vi "Perform Action.vi"(8 "error in":errorcluster, 10 "Input":variant, 11 "HSU MCU V2 in":refnum<class "HSU MCU V2 CFG.lvclass">) -> (0 "error out":errorcluster, 2 "Output":variant, 3 "HSU MCU V2 out":refnum<class "HSU MCU V2 CFG.lvclass">)   [LabVIEW 2023, in "HSU MCU V2 CFG.lvclass"]
uses:
  HSU MCU V2 CFG.lvclass
  Attribute Selector.ctl
  MCU Selector.ctl
  HSU MCU V2 CFG.lvclass/HSU MCU V2 CFG.ctl
  Protocols/ICAN/ICAN.lvclass
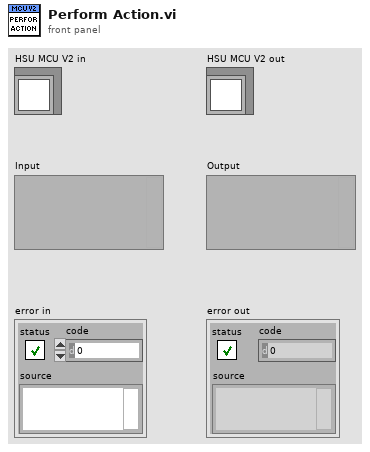
[diagram p1: front panel]
types:
  T1 = typedef "MCU Selector.ctl" = enum16{"Default", "MCU1", "MCU2", "MCU3", "MCU4", "MCU5", "MCU6", "MCU7", "MCU8", "ALL"}
  T2 = typedef "Attribute Selector.ctl" = enum16{"MCU_FAULT", "ALL", "MCU_STATE", "MCU_Temp_Winding", "MCU_Temp_PowerStage", "MCU_Speed", "MCU_I_REF", "MCU_ENABLE", "MCU_U_DC", "Power", "Torque"}
  T3 = cluster{"Action":enum16{"Read", "Write"}, "MCU":string, "Attribute":string, "Value":variant}
  T4 = cluster{"Frame.Signal Names":string[], "Frame.Signal Values":dbl[]}
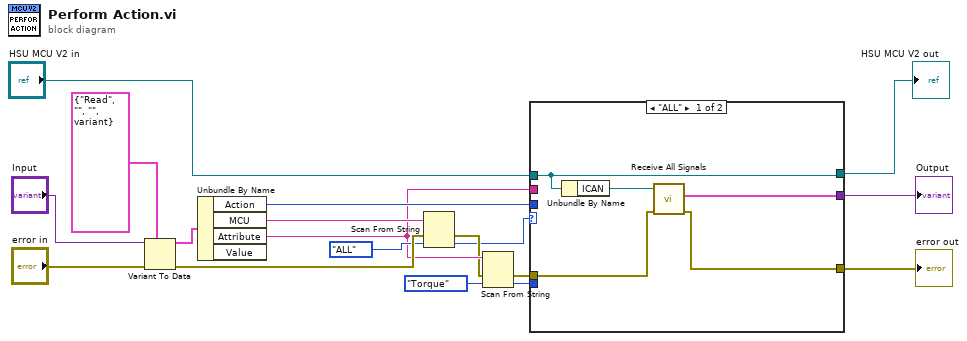
[diagram p0: block diagram]
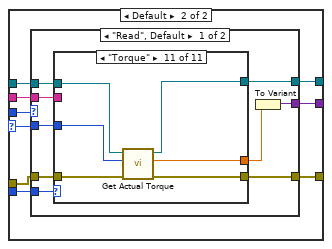
[diagram p2: hidden frame]
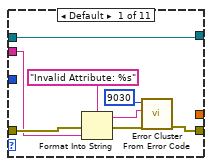
[diagram p3: hidden frame]
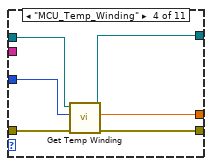
[diagram p6: hidden frame]
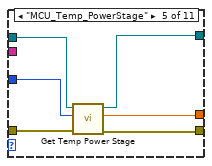
[diagram p7: hidden frame]
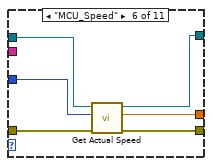
[diagram p8: hidden frame]
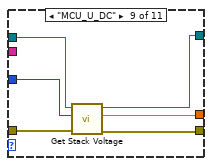
[diagram p11: hidden frame]
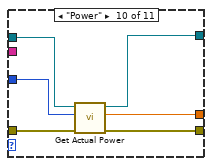
[diagram p12: hidden frame]
diagram:
  n1 = Variant To Data(error in="error in", type=T3 {"Action"=enum."Read", "MCU"="", "Attribute"="", "Value"=variant}, Variant="Input") -> (data=w2:T3, error out=w14:errorcluster)
  n2 = Unbundle By Name(w2) -> ("Action"=w17:enum16{"Read", "Write"}, "MCU"=w7:string, "Attribute"=w5:string)  [unwired: 1 out]
  n3 = Scan From String(input string=w7, error in=w14, default 1=MCU_Selector."ALL" ("MCU Selector")) -> (error out=w4:errorcluster, output 1=w1:T1)  [unwired: 2 in, 2 out]
  n4 = Scan From String(input string=w5, error in=w4, default 1=Attribute_Selector."Torque") -> (error out=w9:errorcluster, output 1=w8:T2)  [unwired: 2 in, 2 out]
  n5 = case shown="\"ALL\"" w1 {
    selector: w1 -> [_ w24]
    tunnel: w17 -> [_ w32]
    tunnel: [w21 w31] -> w16
    tunnel: [w20 w30] -> w13
    tunnel: "HSU MCU V2 in" -> [w19 w29]
    tunnel: [w19 w28] -> w11
    tunnel: w9 -> [w22 w27]
    tunnel: w8 -> [_ w26]
    tunnel: w5 -> [_ w25]
    frame "ALL" {
      n6 = Unbundle By Name(w19) -> ("ICAN"=w23:refnum<class "ICAN.lvclass">)
      n7 = call-dynamic "Receive All Signals.vi"("error in"=w22, "ICAN in"=w23) -> ("error out"=w21:errorcluster, "All Signals"=w20:T4)  [unwired: 7 in, 1 out]
    }
    frame Default {
      n8 = case shown="\"Read\", Default" w32 {
        tunnel: w29 -> [w41 w94]
        tunnel: [w40 w95] -> w31
        tunnel: [w33 _] -> w30
        tunnel: [w38 w94] -> w28
        tunnel: w27 -> [w37 w95]
        tunnel: w26 -> [w36 _]
        tunnel: w24 -> [w35 _]
        tunnel: w25 -> [w34 _]
        frame "Read", Default {
          n9 = case shown="\"Torque\"" w36 {
            tunnel: w37 -> [w46 w50 w53 w59 w65 w71 w72 w74 w81 w87 w93]
            tunnel: w41 -> [w44 w51 w52 w57 w63 w67 w73 w75 w79 w84 w91]
            tunnel: [w49 w50 w53 w54 w60 w70 w72 w74 w78 w86 w92] -> w40
            tunnel: [_ _ _ w55 w61 w68 _ _ w77 w85 w89] -> w39
            tunnel: [w44 w51 w52 w56 w62 w66 w73 w75 w76 w83 w90] -> w38
            tunnel: w35 -> [_ _ _ w58 w64 w69 _ _ w80 w82 w88]
            tunnel: w34 -> [w43 _ _ _ _ _ _ _ _ _ _]
            frame Default {
              n10 = Format Into String(format string="Invalid Attribute: %s" ("error message (\"\")"), error in=w46, w43) -> (resulting string=w48:string, error out=w45:errorcluster)  [unwired: 1 in]
              n11 = call <vilib>:"Error Cluster From Error Code.vi"("error in (no error)"=w45, "error message (\"\")"=w48, "error code (0)"=9030) -> ("error out"=w49:errorcluster)  [unwired: 6 in]
            }
            frame "MCU_FAULT" {
            }
            frame "MCU_STATE" {
            }
            frame "MCU_Temp_Winding" {
              n12 = call "Get Temp Winding.vi"("error in"=w59, 10:w58, "HSU MCU V2 Monitor CFG in"=w57) -> ("error out"=w54:errorcluster, "Temperature"=w55:dbl, "HSU MCU V2 Monitor CFG out"=w56:refnum<class "HSU MCU V2 CFG.lvclass">)  [unwired: 6 in]
            }
            frame "MCU_Temp_PowerStage" {
              n13 = call "Get Temp Power Stage.vi"("error in"=w65, 10:w64, "HSU MCU V2 Monitor CFG in"=w63) -> ("error out"=w60:errorcluster, "Temperature"=w61:dbl, "HSU MCU V2 Monitor CFG out"=w62:refnum<class "HSU MCU V2 CFG.lvclass">)  [unwired: 6 in]
            }
            frame "MCU_Speed" {
              n14 = call "Get Actual Speed.vi"("error in"=w71, 10:w69, "HSU MCU V2 Monitor CFG in"=w67) -> ("error out"=w70:errorcluster, "Speed"=w68:dbl, "HSU MCU V2 Monitor CFG out"=w66:refnum<class "HSU MCU V2 CFG.lvclass">)  [unwired: 6 in]
            }
            frame "MCU_I_REF" {
            }
            frame "MCU_ENABLE" {
            }
            frame "MCU_U_DC" {
              n15 = call "Get Stack Voltage.vi"("error in"=w81, 10:w80, "HSU MCU V2 Monitor CFG in"=w79) -> ("error out"=w78:errorcluster, "Voltage DC"=w77:dbl, "HSU MCU V2 Monitor CFG out"=w76:refnum<class "HSU MCU V2 CFG.lvclass">)  [unwired: 6 in]
            }
            frame "Power" {
              n16 = call "Get Actual Power.vi"("error in"=w87, 10:w82, "HSU MCU V2 CFG in"=w84) -> ("error out"=w86:errorcluster, "Power"=w85:dbl, "HSU MCU V2 CFG out"=w83:refnum<class "HSU MCU V2 CFG.lvclass">)  [unwired: 5 in, 1 out]
            }
            frame "Torque" {
              n17 = call "Get Actual Torque.vi"("error in"=w93, "MCU Selector"=w88, "HSU MCU V2 Monitor CFG in"=w91) -> ("error out"=w92:errorcluster, "Torque"=w89:dbl, "HSU MCU V2 Monitor CFG out"=w90:refnum<class "HSU MCU V2 CFG.lvclass">)  [unwired: 6 in]
            }
          }
          n18 = To Variant(anything=w39) -> (Variant=w33:variant)
        }
        frame "Write" {
        }
      }
    }
  }
  "error out" <- w16
  "HSU MCU V2 out" <- w11
  "Output" <- w13
